vi "Get Water Level.vi"(8 "error in (no error)":errorcluster, 11 "HW Water Level in":refnum<class "HW Water Level.lvclass">) -> (0 "error out":errorcluster, 2 "Water Level":dbl)   [LabVIEW 2018, in "HW Water Level.lvclass"]
uses:
  HW Water Level.lvclass
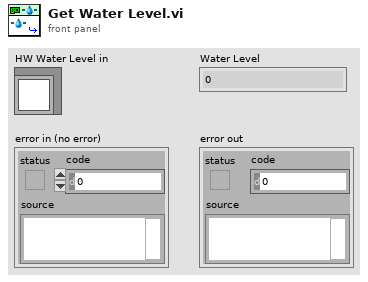
[diagram p1: front panel]
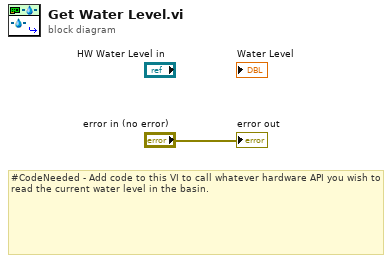
[diagram p0: block diagram]
diagram:
  # "#CodeNeeded - Add code to this VI to call whatever hardware API you wish to read the current water level in the basin."
  "error out" <- "error in (no error)"
